vi "Document My VI - Set Review Date.vi"(8 "error in (no error)":errorcluster) -> (0 "error out":errorcluster, 2 "Canceled":bool, 3 "Date of Review out":timestamp=timestamp(3345454800 s since 1904-01-01) format="%<%m/%d/%Y>T")   [LabVIEW 2014]
panel:
  in  "Set No Review":bool
  in  "OK":bool
  in  "Date of Review":timestamp=timestamp(3345454800 s since 1904-01-01) format="%<%m/%d/%Y>T"
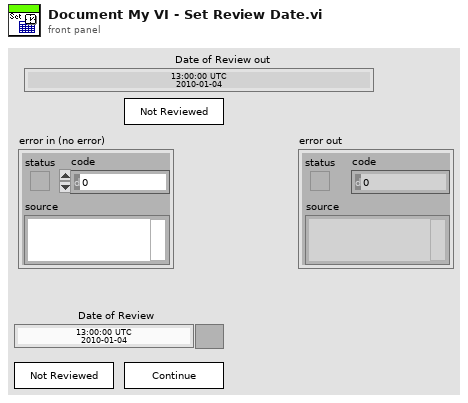
[diagram p1: front panel]
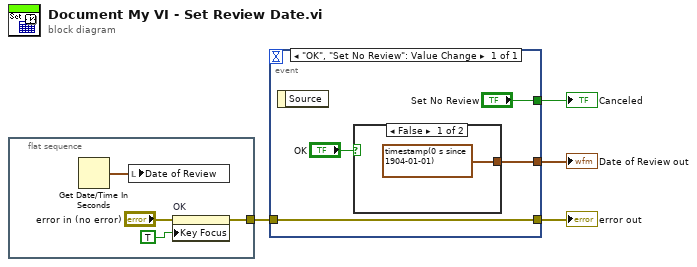
[diagram p0: block diagram]
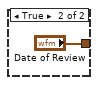
[diagram p2: hidden frame]
diagram:
  n1 = flat-sequence {
    tunnel: [w5] -> w4
    frame #0 {
      n2 = Get Date/Time In Seconds() -> (seconds since 1Jan1904=w8:timestamp)
      n3 = local write "Date of Review"(w8) -> ()
      n4 = property on="OK" class="Bool"(error in="error in (no error)", "Key Focus"=TRUE) -> (error out=w5:errorcluster)  [unwired: 1 in, 1 out]
    }
  }
  n5 = event shown="[0] \"OK\", \"Set No Review\": Value Change" {
    selector: _ -> [_]
    dyn-events: _ -> [_]
    timeout: _ -> [_]
    tunnel: w4 -> [w10]
    tunnel: [w11] -> w3
    tunnel: [w10] -> w2
    tunnel: ["Set No Review"] -> w1
    event "OK", "Set No Review": Value Change {
      n6 = event-data() -> ()  [unwired: 1 in, 1 out]
      n7 = case shown="False" "OK" {
        tunnel: [timestamp(0 s since 1904-01-01) ("Date of Review") "Date of Review"] -> w11
        frame False {
        }
        frame True {
        }
      }
    }
  }
  "error out" <- w2
  "Date of Review out" <- w3
  "Canceled" <- w1
